vi "Connect.vi"(8 "error in (no error)":errorcluster, 10 "Connection":T1 {"Custom Data" format="%.0x"}, 11 "CIFTag in":refnum<class "CIF_CIPC_Chn.lvclass">) -> (0 "error out":errorcluster, 3 "CIFTag out":refnum<class "CIF_CIPC_Chn.lvclass">)   [LabVIEW 2021, in "CIF_CIPC_Chn.lvclass"]
uses:
  CIF_CIPC_Chn.lvclass
  D:/dev/Packages/CIF_Channels_Core/src/CIFChannels/CIFChannels.lvclass
  CIFChannels/CIFChannels.lvclass/CIFChannels.ctl
  CIFChannels/Typedef/Channel State.ctl
  CIF_CIPC_Chn.lvclass/CIF_CIPC_Chn.ctl
  CIFChannels/Accessors/Read Direction.vi
  <vilib>/CIF Foundation/CIF Utilities/DataTypes/Flatten Unflatten/Unflatten U32.vi
  <vilib>/CIF Foundation/CIF Utilities/DataTypes/Flatten Unflatten/Unflatten I32.vi
  <vilib>/CIF Foundation/CIF Utilities/DataTypes/Flatten Unflatten/Unflatten U64.vi
  <vilib>/CIF Foundation/CIF CIPC/SubVIs/Check Error.vi
  <vilib>/CIF Foundation/CIF CIPC/SubVIs/Get dll Path.vi
  <vilib>/CIF Foundation/CIF CIPC/Utilities/Decode Data Element Descriptions.vi
  <vilib>/Utility/error.llb/Trim Whitespace.vi
  <vilib>/Utility/error.llb/Error Cluster From Error Code.vi
  CIFChannels/CIFChannels.lvclass
  <vilib>/CIF Foundation/CIF CIPC/CIF_NI_CIPC.lvlib
  D:/dev/Packages/CIF_Channels_Core/src/CIPC_Channels/CIF_CIPC_Chan/CIF_CIPC_Chn.lvclass
  ChannelCommon/typedef/New FIFO Instance Response.ctl
  ChannelCommon/ChannelCommon.lvlib
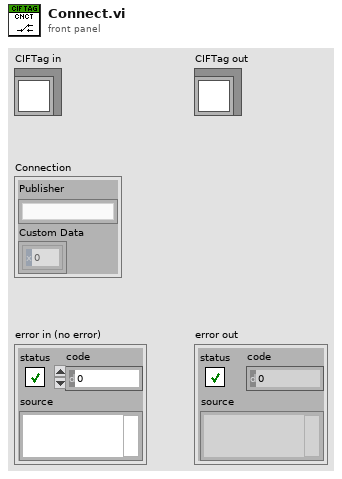
[diagram p1: front panel]
types:
  T1 = typedef "ChannelCommon.lvlib/New FIFO Instance Response.ctl" = cluster{"Publisher":string, "Custom Data":u8[]}
  T2 = typedef "CIFChannels.lvclass/Channel State.ctl" = enum16{"Creating", "Disconnected", "Connecting", "Connected", "Destroyed"}
  T3 = typedef "CIFChannels.lvclass/Direction.ctl" = enum16{"Publisher", "Subscriber"}
  T4 = typedef "CIF_CIPC_Chn.lvclass/Buffer Configuration Data.ctl" = cluster{"Total Size":u32, "Read Size":u32, "Read Offset":u32, "CIPC BP References":T5, "Override CIPC Name":string, "Encoder Data":string}
  T5 = typedef "CIF_NI_CIPC.lvlib/Backpressure References.ctl" = cluster{"CIPC Reference":u64, "CIPC BP Reference":u64}
  T6 = typedef "CIF_NI_CIPC.lvlib/Encoder Info.ctl" = cluster{"Name":string, "Version":i32, "Data":string}
  T7 = typedef "NI_Data Type.lvlib/Data Type.ctl" = enum8{"Invalid Type", "Void", "I8", "I16", "I32", "I64", "U8", "U16", "U32", "U64", "Single Float", "Double Float", "Extended Float", "Single Complex", "Double Complex", "Extended Complex", "Enum U8", "Enum U16", "Enum U32", "Enum U64", "Single Float With Unit", "Double Float With Unit", "Extended Float With Unit", "Single Complex with Unit", "Double Complex with Unit", "Extended Complex with Unit", "Boolean", "String", "Path", "Picture", "Tag", "Array", "Cluster", "Variant", "LV Variant", "Waveform", "Timestamp", "Digital Waveform", "Digital Data", "ExpressData", "Refnum", "External Data", "VI", "Poly VI", "LabVIEW Class Instance", "Fixed Point", "Set Collection", "Map Collection"}
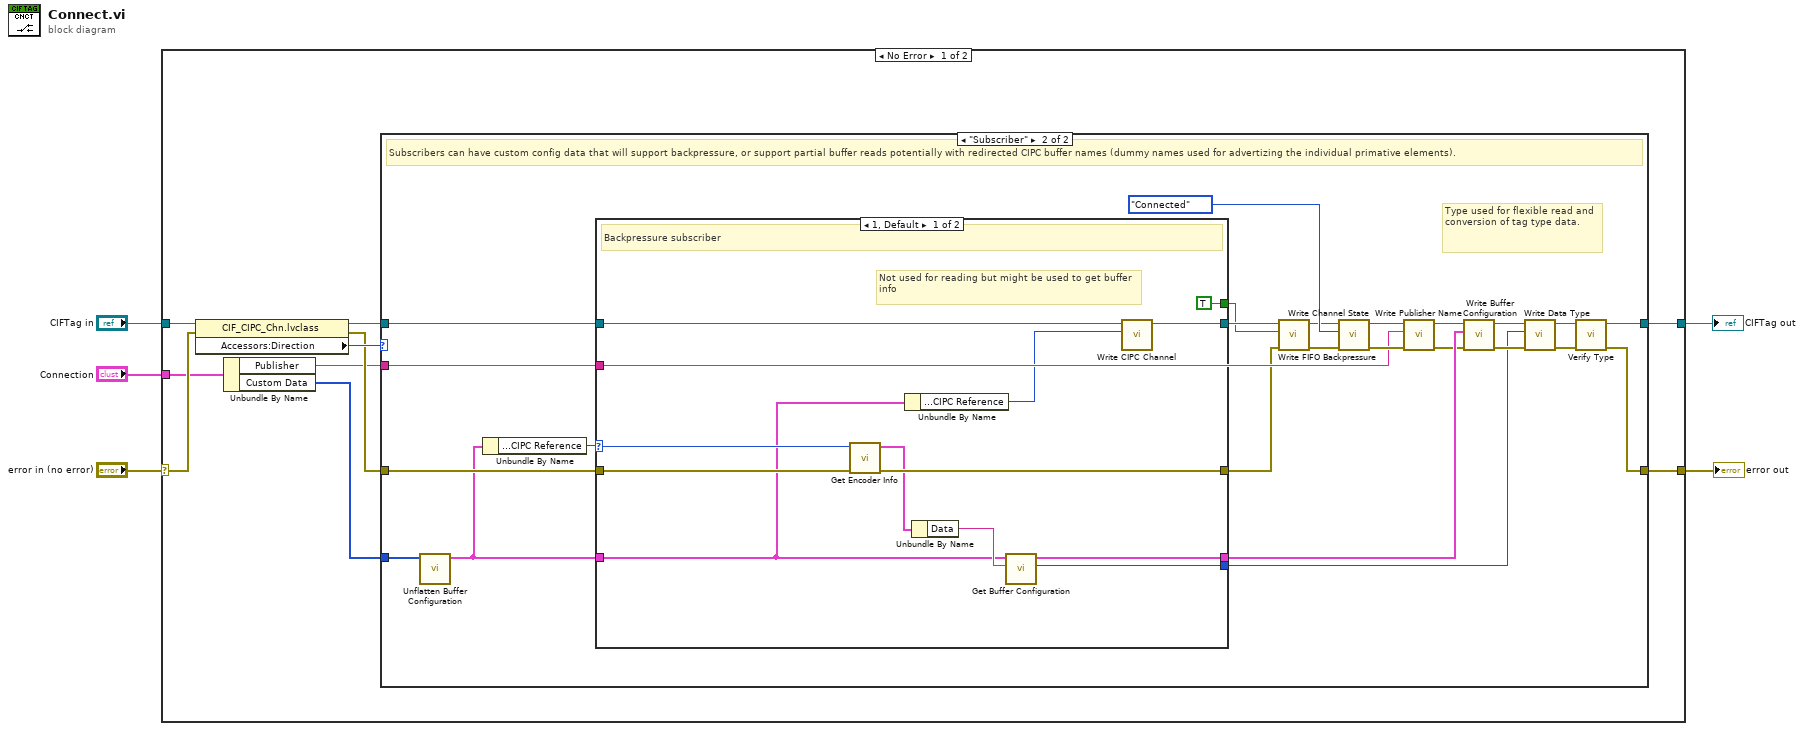
[diagram p0: block diagram]
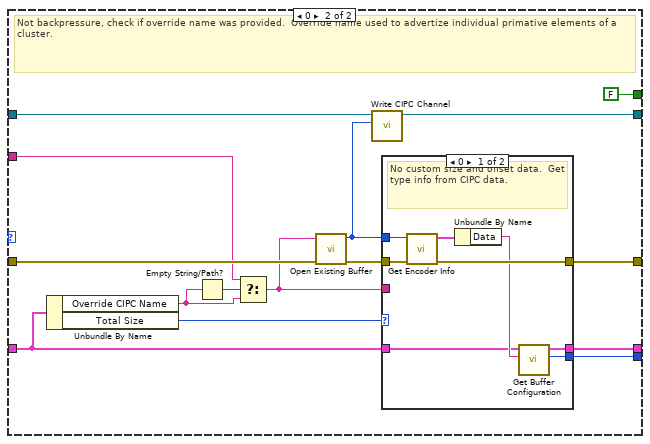
[diagram p3: hidden frame]
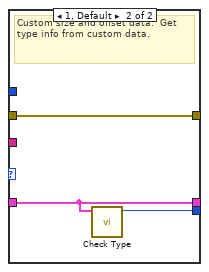
[diagram p4: hidden frame]
diagram:
  n1 = case shown="No Error" "error in (no error)" {
    selector: "error in (no error)" -> [w14 w81]
    tunnel: [w9 w81] -> w4
    tunnel: [w11 w80] -> w2
    tunnel: "CIFTag in" -> [w15 w80]
    tunnel: "Connection" -> [w8 _]
    frame No Error {
      n2 = property class="CIF_CIPC_Chn.lvclass"(reference=w15, error in=w14) -> (reference out=w13:refnum<class "CIF_CIPC_Chn.lvclass">, error out=w10:errorcluster, "Accessors:Direction"=w12:T3)
      n3 = Unbundle By Name(w8) -> ("Publisher"=w7:string, "Custom Data"=w6:u8[])
      n4 = case shown="\"Subscriber\"" w12 {
        tunnel: w13 -> [w17 w26]
        tunnel: [w17 w31] -> w11
        tunnel: w10 -> [w16 w38]
        tunnel: w7 -> [_ w27]
        tunnel: [w16 w30] -> w9
        tunnel: w6 -> [_ w29]
        frame "Publisher" {
          # "No connection step needed for publishers"
        }
        frame "Subscriber" {
          # "Type used for flexible read and conversion of tag type data."
          # "Subscribers can have custom config data that will support backpressure, or support partial buffer reads potentially with redirected CIPC buffer names (dummy names used for advertizing the individual primative elements)."
          n5 = call "Unflatten Buffer Configuration.vi"("Flattened Configuration"=w29) -> ("Buffer Configuration"=w28:T4)  [unwired: 10 in]
          n6 = Unbundle By Name(w28) -> ("CIPC BP References.CIPC Reference"=w23:u64)
          n7 = case shown="1, Default" w23 {
            selector: w23 -> [w53 _]
            tunnel: w38 -> [w52 w68]
            tunnel: [w50 w67] -> w37
            tunnel: [w49 w66] -> w34
            tunnel: w28 -> [w43 w61]
            tunnel: w27 -> [_ w60]
            tunnel: w26 -> [w46 w58]
            tunnel: [w45 w57] -> w21
            tunnel: [w51 w55] -> w22
            tunnel: [TRUE ("Backpressure") FALSE ("Backpressure")] -> w18
            frame 1, Default {
              # "Not used for reading but might be used to get buffer info"
              # "Backpressure subscriber"
              n8 = call <vilib>:"Get Encoder Info.vi"("error in (no error)"=w52, "CIPC Reference"=w53) -> ("error out"=w51:errorcluster, "Encoder Info"=w44:T6)  [unwired: 8 in]
              n9 = Unbundle By Name(w43) -> ("CIPC BP References.CIPC Reference"=w42:u64)
              n10 = Unbundle By Name(w44) -> ("Data"=w48:string)
              n11 = call "Get Buffer Configuration.vi"("Encoder Data Description"=w48, "Buffer Configuration in"=w43) -> ("Type"=w49:T7, "Buffer Configuration out"=w50:T4)  [unwired: 8 in]
              n12 = call "Write CIPC Channel.vi"("CIF Channel"=w42, "CIFTag in"=w46) -> ("CIFTag out"=w45:refnum<class "CIF_CIPC_Chn.lvclass">)  [unwired: 8 in, 1 out]
            }
            frame 0 {
              # "Not backpressure, check if override name was provided.  Override name used to advertize individual primative elements of a cluster."
              n13 = Unbundle By Name(w61) -> ("Override CIPC Name"=w64:string, "Total Size"=w63:u32)
              n14 = Empty String/Path?(string/path=w64) -> (empty?=w65:bool)
              n15 = Select(t=w60, s=w65, f=w64) -> (s? t:f=w62:string)
              n16 = call <vilib>:"Open Existing Buffer.vi"("error in (no error)"=w68, "buffer_name"=w62) -> ("error out"=w56:errorcluster, "CIPC Reference"=w59:u64)  [unwired: 8 in]
              n17 = call "Write CIPC Channel.vi"("CIF Channel"=w59, "CIFTag in"=w58) -> ("CIFTag out"=w57:refnum<class "CIF_CIPC_Chn.lvclass">)  [unwired: 8 in, 1 out]
              n18 = case shown="0" w63 {
                tunnel: [w74 w78] -> w67
                tunnel: w59 -> [w76 _]
                tunnel: [w73 w79] -> w66
                tunnel: w61 -> [w69 w78]
                tunnel: w62 -> [_ _]
                tunnel: w56 -> [w72 w77]
                tunnel: [w71 w77] -> w55
                frame 0 {
                  # "No custom size and offset data.  Get type info from CIPC data."
                  n19 = call <vilib>:"Get Encoder Info.vi"("error in (no error)"=w72, "CIPC Reference"=w76) -> ("error out"=w71:errorcluster, "Encoder Info"=w75:T6)  [unwired: 8 in]
                  n20 = Unbundle By Name(w75) -> ("Data"=w70:string)
                  n21 = call "Get Buffer Configuration.vi"("Encoder Data Description"=w70, "Buffer Configuration in"=w69) -> ("Type"=w73:T7, "Buffer Configuration out"=w74:T4)  [unwired: 8 in]
                }
                frame 1, Default {
                  # "Custom size and offset data.  Get type info from custom data."
                  n22 = call "Check Type.vi"("Buffer Configuration"=w78) -> ("Type"=w79:T7)  [unwired: 10 in]
                }
              }
            }
          }
          n23 = call "Write FIFO Backpressure.vi"("error in (no error)"=w22, "Backpressure"=w18, "CIFChannels in"=w21) -> ("error out"=w20:errorcluster, "CIFChannels out"=w19:refnum<class "CIF_CIPC_Chn.lvclass">)  [unwired: 7 in]
          n24 = call "Write Channel State.vi"("error in (no error)"=w20, "Channel State"=Channel_State."Connected", "CIFChannels in"=w19) -> ("error out"=w39:errorcluster, "CIFChannels out"=w40:refnum<class "CIF_CIPC_Chn.lvclass">)  [unwired: 7 in]
          n25 = call "Write Publisher Name.vi"("error in (no error)"=w39, "Publisher Name"=w27, "CIFChannels in"=w40) -> ("error out"=w25:errorcluster, "CIFChannels out"=w24:refnum<class "CIF_CIPC_Chn.lvclass">)  [unwired: 7 in]
          n26 = call "Write Buffer Configuration.vi"("error in (no error)"=w25, "Buffer Configuration"=w37, "CIF_CIPC_Chn in"=w24) -> ("error out"=w35:errorcluster, "CIF_CIPC_Chn out"=w36:refnum<class "CIF_CIPC_Chn.lvclass">)  [unwired: 7 in]
          n27 = call "Write Data Type.vi"("error in (no error)"=w35, "Type Enum"=w34, "CIF_CIPC_Chn in"=w36) -> ("error out"=w32:errorcluster, "CIF_CIPC_Chn out"=w33:refnum<class "CIF_CIPC_Chn.lvclass">)  [unwired: 7 in]
          n28 = call-dynamic "Verify Type.vi"("error in (no error)"=w32, "CIF_CIPC_Chn in"=w33) -> ("error out"=w30:errorcluster, "CIF_CIPC_Chn out"=w31:refnum<class "CIF_CIPC_Chn.lvclass">)  [unwired: 8 in]
        }
      }
    }
    frame Error {
    }
  }
  "error out" <- w4
  "CIFTag out" <- w2
